vi "CalcTemperature.vi"(11 "Array":string[](array[string])) -> (3 "HJ Temperature (°C)":dbl)   [LabVIEW 2024]
panel:
  out "CJ Temperature (°C)":dbl
  out "Junction Delta Temperature (°C)":dbl
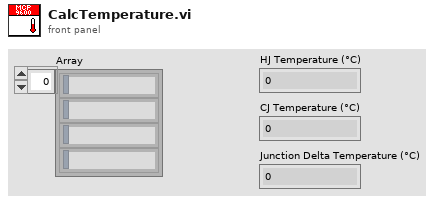
[diagram p1: front panel]
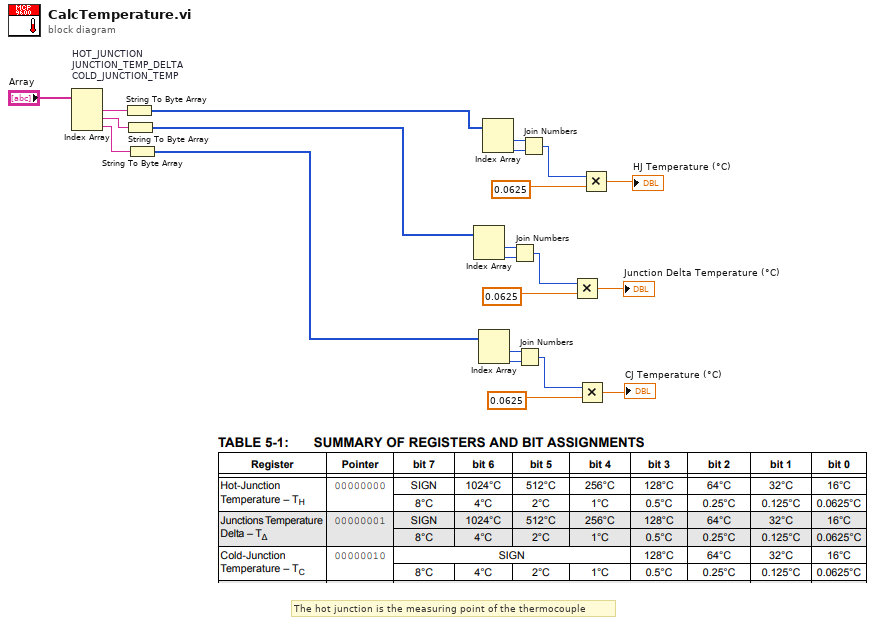
[diagram p0: block diagram]
diagram:
  # "The hot junction is the measuring point of the thermocouple"
  n1 = Index Array "HOT_JUNCTION\nJUNCTION_TEMP_DELTA\nCOLD_JUNCTION_TEMP"(array="Array") -> (element #1=w20:string, element #2=w19:string, element #3=w18:string)  [unwired: 3 in]
  n2 = String To Byte Array(string=w20) -> (unsigned byte array=w22:u8[])
  n3 = String To Byte Array(string=w19) -> (unsigned byte array=w4:u8[])
  n4 = String To Byte Array(string=w18) -> (unsigned byte array=w3:u8[])
  n5 = Index Array(array=w4) -> (element #1=w9:u8, element #2=w10:u8)  [unwired: 2 in]
  n6 = Index Array(array=w3) -> (element #1=w8:u8, element #2=w7:u8)  [unwired: 2 in]
  n7 = Index Array(array=w22) -> (element #1=w17:u8, element #2=w16:u8)  [unwired: 2 in]
  n8 = Join Numbers(hi=w9, lo=w10) -> ((hi.lo)=w11:u16)
  n9 = Join Numbers(hi=w8, lo=w7) -> ((hi.lo)=w6:u16)
  n10 = Join Numbers(hi=w17, lo=w16) -> ((hi.lo)=w15:u16)
  n11 = Multiply(x=w11, y=0.0625) -> (x*y=→"Junction Delta Temperature (°C)":dbl)
  n12 = Multiply(x=w6, y=0.0625) -> (x*y=→"CJ Temperature (°C)":dbl)
  n13 = Multiply(x=w15, y=0.0625) -> (x*y=→"HJ Temperature (°C)":dbl)
